vi "initialiseStartValue.vi"(8 "error in (no error)":errorcluster, 11 "ScanCreator in":refnum<class "ScanCreator.lvclass">) -> (0 "error out":errorcluster, 3 "ScanCreator out":refnum<class "ScanCreator.lvclass">)   [LabVIEW 2011, in "Views.lvlib" / "ScriptEditor.lvlib" / "ScanCreator.lvclass"]
uses:
  ScanCreator.lvclass
  ScanCreator.lvclass/ScanCreator.ctl
  Tools/Scripting/ScriptingEvent/ScriptEvents/Ramp/RampEvent/RampEvent.lvclass
  Tools/Scripting/ScriptingEvent/ScriptEvents/Rf Event/rf.lvclass
  Tools/Scripting/ScriptingEvent/ScriptEvent.lvclass
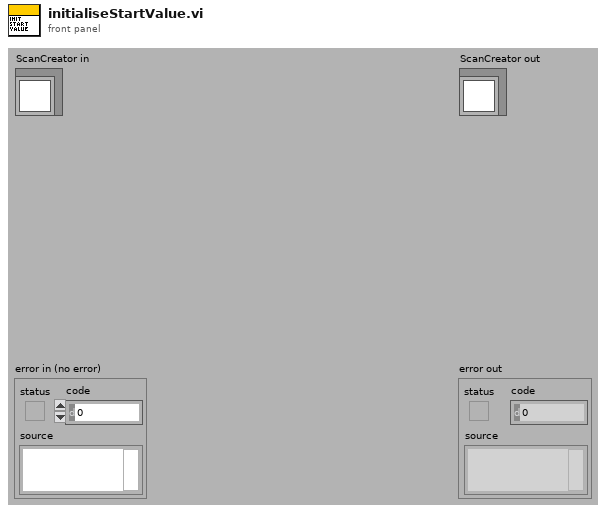
[diagram p1: front panel]
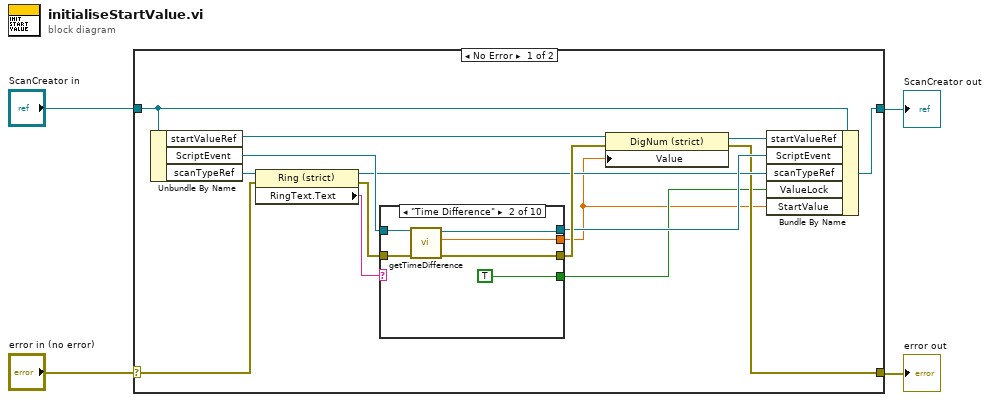
[diagram p0: block diagram]
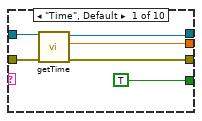
[diagram p2: hidden frame]
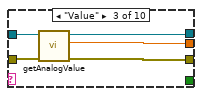
[diagram p3: hidden frame]
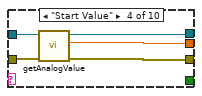
[diagram p4: hidden frame]
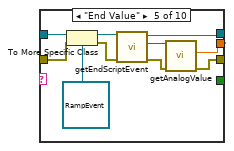
[diagram p5: hidden frame]
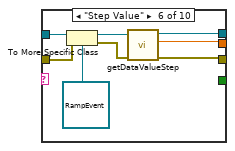
[diagram p6: hidden frame]
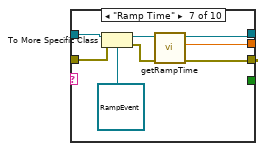
[diagram p7: hidden frame]
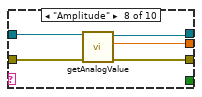
[diagram p8: hidden frame]
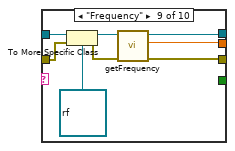
[diagram p9: hidden frame]
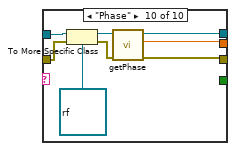
[diagram p10: hidden frame]
diagram:
  n1 = case shown="No Error" "error in (no error)" {
    selector: "error in (no error)" -> [w15 w90]
    tunnel: [w8 w90] -> w3
    tunnel: [w6 w89] -> w1
    tunnel: "ScanCreator in" -> [w12 w89]
    frame No Error {
      n2 = Unbundle By Name(w12) -> ("startValueRef"=w14:refnum<vi>, "ScriptEvent"=w17:refnum<class "ScriptEvent.lvclass">, "scanTypeRef"=w19:refnum<vi>)
      n3 = property class="Ring (strict)"(reference=w19, error in=w15) -> (reference out=w9:refnum<vi>, error out=w16:errorcluster, "RingText.Text"=w18:string)
      n4 = case shown="\"Time Difference\"" w18 {
        tunnel: w17 -> [w25 w31 w36 w41 w51 w58 w66 w72 w80 w87]
        tunnel: w16 -> [w24 w30 w35 w40 w49 w57 w65 w69 w79 w86]
        tunnel: [w23 w28 w34 w39 w43 w53 w61 w70 w74 w82] -> w5
        tunnel: [w22 w27 w32 w37 w42 w52 w60 w68 w73 w81] -> w13
        tunnel: [w21 w29 w33 w38 w44 w54 w62 w71 w75 w83] -> w10
        tunnel: [TRUE TRUE _ _ _ _ _ _ _ _] -> w7
        frame "Time", Default {
          n5 = call "getTime.vi"("error in (no error)"=w24, "ScriptEvent.lvclass in"=w25) -> ("error out"=w22:errorcluster, "time"=w23:dbl, "ScriptEvent.lvclass out"=w21:refnum<class "ScriptEvent.lvclass">)  [unwired: 7 in]
        }
        frame "Time Difference" {
          n6 = call "getTimeDifference.vi"("error in (no error)"=w30, "ScriptEvent.lvclass in"=w31) -> ("error out"=w27:errorcluster, "time difference"=w28:dbl, "ScriptEvent.lvclass out"=w29:refnum<class "ScriptEvent.lvclass">)  [unwired: 7 in]
        }
        frame "Value" {
          n7 = call "getAnalogValue.vi"("error in (no error)"=w35, "ScriptEvent in"=w36) -> ("error out"=w32:errorcluster, "analogValue"=w34:dbl, "ScriptEvent out"=w33:refnum<class "ScriptEvent.lvclass">)  [unwired: 7 in]
        }
        frame "Start Value" {
          n8 = call "getAnalogValue.vi"("error in (no error)"=w40, "ScriptEvent in"=w41) -> ("error out"=w37:errorcluster, "analogValue"=w39:dbl, "ScriptEvent out"=w38:refnum<class "ScriptEvent.lvclass">)  [unwired: 7 in]
        }
        frame "End Value" {
          n9 = To More Specific Class(target class=refnum<class "RampEvent.lvclass"> refnum ("Tools.lvlib:Scripting.lvlib:RampEvent.lvclass"), reference=w51, error in=w49) -> (specific class reference=w48:refnum<class "RampEvent.lvclass">, error out=w47:errorcluster)
          n10 = call "getEndScriptEvent.vi"("error in (no error)"=w47, "RampEvent.lvclass in"=w48) -> ("error out"=w45:errorcluster, "ScriptEvent.lvclass"=w46:refnum<class "ScriptEvent.lvclass">, "RampEvent.lvclass out"=w44:refnum<class "RampEvent.lvclass">)  [unwired: 7 in]
          n11 = call "getAnalogValue.vi"("error in (no error)"=w45, "ScriptEvent in"=w46) -> ("error out"=w42:errorcluster, "analogValue"=w43:dbl)  [unwired: 7 in, 1 out]
        }
        frame "Step Value" {
          n12 = To More Specific Class(target class=refnum<class "RampEvent.lvclass"> refnum ("Tools.lvlib:Scripting.lvlib:RampEvent.lvclass"), reference=w58, error in=w57) -> (specific class reference=w56:refnum<class "RampEvent.lvclass">, error out=w55:errorcluster)
          n13 = call-dynamic "getDataValueStep.vi"("error in (no error)"=w55, "RampEvent.lvclass in"=w56) -> ("error out"=w52:errorcluster, "dataValueStep"=w53:dbl, "RampEvent.lvclass out"=w54:refnum<class "RampEvent.lvclass">)  [unwired: 7 in]
        }
        frame "Ramp Time" {
          n14 = To More Specific Class(target class=refnum<class "RampEvent.lvclass"> refnum ("Tools.lvlib:Scripting.lvlib:RampEvent.lvclass"), reference=w66, error in=w65) -> (specific class reference=w64:refnum<class "RampEvent.lvclass">, error out=w63:errorcluster)
          n15 = call "getRampTime.vi"("error in (no error)"=w63, "RampEvent.lvclass in"=w64) -> ("error out"=w60:errorcluster, "rampTime"=w61:dbl, "RampEvent.lvclass out"=w62:refnum<class "RampEvent.lvclass">)  [unwired: 7 in]
        }
        frame "Amplitude" {
          n16 = call "getAnalogValue.vi"("error in (no error)"=w69, "ScriptEvent in"=w72) -> ("error out"=w68:errorcluster, "analogValue"=w70:dbl, "ScriptEvent out"=w71:refnum<class "ScriptEvent.lvclass">)  [unwired: 7 in]
        }
        frame "Frequency" {
          n17 = To More Specific Class(target class=refnum<class "rf.lvclass"> refnum ("Tools.lvlib:Scripting.lvlib:rf.lvclass"), reference=w80, error in=w79) -> (specific class reference=w77:refnum<class "rf.lvclass">, error out=w76:errorcluster)
          n18 = call "getFrequency.vi"("error in (no error)"=w76, "rf in"=w77) -> ("error out"=w73:errorcluster, "frequency"=w74:dbl, "rf out"=w75:refnum<class "rf.lvclass">)  [unwired: 7 in]
        }
        frame "Phase" {
          n19 = To More Specific Class(target class=refnum<class "rf.lvclass"> refnum ("Tools.lvlib:Scripting.lvlib:rf.lvclass"), reference=w87, error in=w86) -> (specific class reference=w85:refnum<class "rf.lvclass">, error out=w84:errorcluster)
          n20 = call "getPhase.vi"("error in (no error)"=w84, "rf in"=w85) -> ("error out"=w81:errorcluster, "phase"=w82:dbl, "rf out"=w83:refnum<class "rf.lvclass">)  [unwired: 7 in]
        }
      }
      n21 = property class="DigNum (strict)"(reference=w14, error in=w13, "Value"=w5) -> (reference out=w11:refnum<vi>, error out=w8:errorcluster)
      n22 = Bundle By Name(cluster=w12, "startValueRef"=w11, "ScriptEvent"=w10, "scanTypeRef"=w9, "ValueLock"=w7, "StartValue"=w5) -> (w6:refnum<class "ScanCreator.lvclass">)
    }
    frame Error {
    }
  }
  "error out" <- w3
  "ScanCreator out" <- w1
